vi "SUPPORTFileInitialization.vi"(11 "Camera Info":T4) -> (0 "AutonArray":dbl[][](array[numeric]), 1 "Current Auton File":string, 2 "ShooterArray":dbl[][](array[numeric]) format="%0.3f", 3 "ShooterFile":string, 4 "Number of Auton Files":i64, 5 "Auton Files":string[](array[string]))   [LabVIEW 2011]
uses:
  <vilib>/Rock Robotics/WPI/Camera/WPI_CameraImageSize.ctl
  <vilib>/Rock Robotics/WPI/Camera/WPI_CameraWhite Balance Values.ctl
  <vilib>/Rock Robotics/WPI/Camera/WPI_CameraExposure Values.ctl
  <vilib>/Utility/file.llb/Read From Spreadsheet File (DBL).vi
panel:
  out "Path and file":string
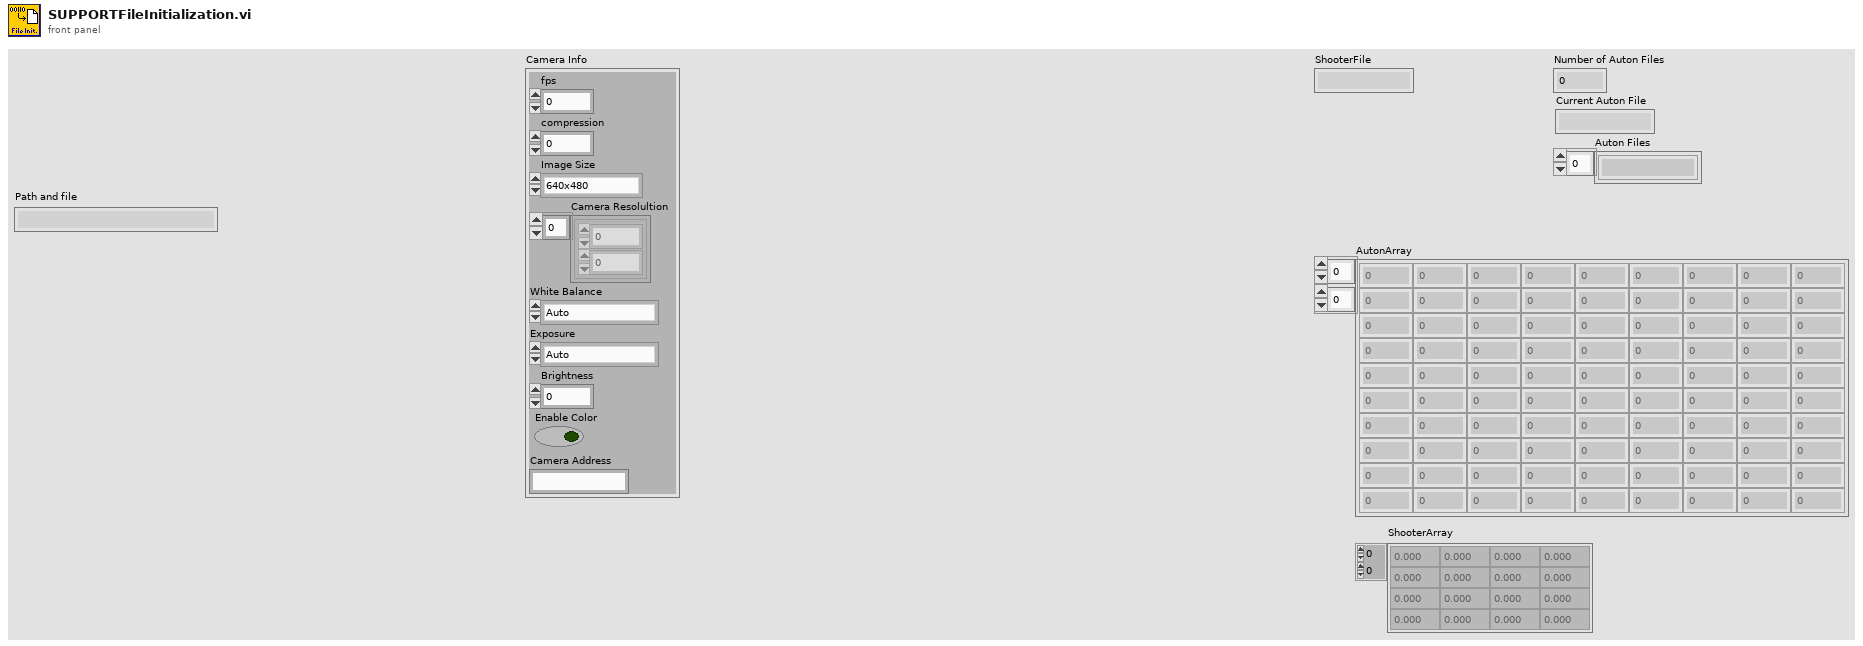
[diagram p1: front panel]
types:
  T1 = typedef "WPI_CameraImageSize.ctl" = enum16{"640x480", "320x240", "160x120"}
  T2 = typedef "WPI_CameraWhite Balance Values.ctl" = enum16{"Auto", "Fixed indoor", "Fixed outdoor 1", "Fixed outdoor 2", "Fixed fluorescent 1", "Fixed fluorescent 2", "Hold current"}
  T3 = typedef "WPI_CameraExposure Values.ctl" = enum16{"Auto", "Flicker-free 50 Hz", "Flicker-free 60 Hz", "Hold current"}
  T4 = cluster{"fps":i32, "compression":i32, "Image Size":T1, "Camera Resolultion":cluster{i32, i32}[], "White Balance":T2, "Exposure":T3, "Brightness":dbl, "Enable Color":bool, "Camera Address":string}
  T5 = typedef "WPI_CameraDevRef.ctl" = cluster{"Camera Address":string, "CameraStatus":errorcluster, "Acquire Image Notifier":refnum<notifier>}
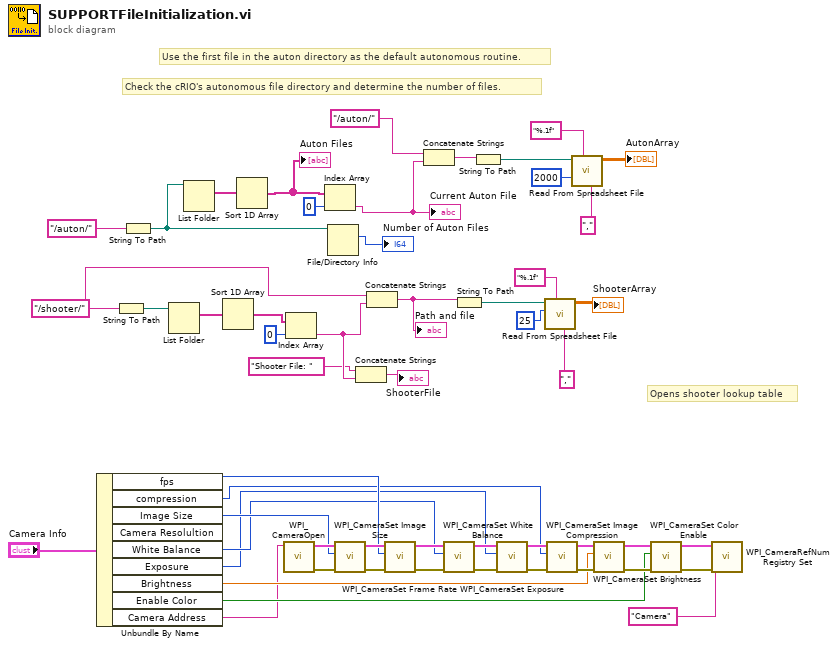
[diagram p0: block diagram]
diagram:
  w19 = "/shooter/" ("string")
  # "Check the cRIO's autonomous file directory and determine the number of files."
  # "Use the first file in the auton directory as the default autonomous routine."
  # "Opens shooter lookup table"
  n1 = Unbundle By Name("Camera Info") -> ("fps"=w37:i32, "compression"=w34:i32, "Image Size"=w38:T1, "White Balance"=w36:T2, "Exposure"=w35:T3, "Brightness"=w33:dbl, "Enable Color"=w32:bool, "Camera Address"=w31:string)  [unwired: 1 out]
  n2 = String To Path(string=w19) -> (path=w28:path)
  n3 = String To Path(string="/auton/") -> (path=w12:path)
  n4 = List Folder(path=w28) -> (filenames=w27:string[])  [unwired: 1 in, 5 out]
  n5 = List Folder(path=w12) -> (filenames=w11:string[])  [unwired: 1 in, 5 out]
  n6 = Sort 1D Array(array=w27) -> (sorted array=w26:string[])
  n7 = Sort 1D Array(array=w11) -> (sorted array=w9:string[])
  "Auton Files" <- w9
  n8 = call <vilib>:"WPI_CameraOpen.vi"("Camera Address"=w31) -> ("error out"=w45:errorcluster, "CameraDevRef"=w44:T5)  [unwired: 1 in, 8 out]
  n9 = Index Array(array=w26, index=0) -> (element=w18:string)
  n10 = Index Array(array=w9, index=0) -> (element=w1:string)
  "Current Auton File" <- w1
  n11 = File/Directory Info(path=w12) -> (size=→"Number of Auton Files":i64)  [unwired: 1 in, 6 out]
  n12 = call <vilib>:"WPI_CameraSet Image Size.vi"("error in (no error)"=w45, "Image Size"=w38, "CameraDevRef"=w44) -> ("error out"=w46:errorcluster, "CameraDevRef Out"=w43:T5)  [unwired: 7 out]
  n13 = Concatenate Strings("Shooter File: ", w18) -> (→"ShooterFile":string)
  n14 = Concatenate Strings(w19, w18) -> (w21:string)
  "Path and file" <- w21
  n15 = call <vilib>:"WPI_CameraSet Frame Rate.vi"("error in (no error)"=w46, "Frame Rate (fps)"=w37, "CameraDevRef"=w43) -> ("error out"=w47:errorcluster, "CameraDevRef Out"=w41:T5)  [unwired: 7 out]
  n16 = Concatenate Strings("/auton/" ("string"), w1) -> (w5:string)
  n17 = call <vilib>:"WPI_CameraSet White Balance.vi"("error in (no error)"=w47, "White Balance"=w36, "CameraDevRef"=w41) -> ("error out"=w48:errorcluster, "CameraDevRef Out"=w42:T5)  [unwired: 7 out]
  n18 = String To Path(string=w21) -> (path=w20:path)
  n19 = String To Path(string=w5) -> (path=w4:path)
  n20 = call <vilib>:"WPI_CameraSet Exposure.vi"("error in (no error)"=w48, "Exposure"=w35, "CameraDevRef"=w42) -> ("error out"=w49:errorcluster, "CameraDevRef Out"=w39:T5)  [unwired: 7 out]
  n21 = call-poly <vilib>:"Read From Spreadsheet File.vi"("delimiter (\\t)"="," ("delimiter (\\t)"), "format (%.3f)"="%.1f", "number of rows (all:-1)"=25, "file path (dialog if empty)"=w20) -> ("all rows"=→"ShooterArray":dbl[][])  [unwired: 1 in, 6 out]
  n22 = call <vilib>:"WPI_CameraSet Image Compression.vi"("error in (no error)"=w49, "Compression"=w34, "CameraDevRef"=w39) -> ("error out"=w50:errorcluster, "CameraDevRef Out"=w40:T5)  [unwired: 7 out]
  n23 = call-poly <vilib>:"Read From Spreadsheet File.vi"("delimiter (\\t)"="," ("delimiter (\\t)"), "format (%.3f)"="%.1f", "number of rows (all:-1)"=2000, "file path (dialog if empty)"=w4) -> ("all rows"=→"AutonArray":dbl[][])  [unwired: 1 in, 6 out]
  n24 = call <vilib>:"WPI_CameraSet Brightness.vi"("error in (no error)"=w50, "Brightness"=w33, "CameraDevRef"=w40) -> ("error out"=w52:errorcluster, "CameraDevRef Out"=w51:T5)  [unwired: 7 out]
  n25 = call <vilib>:"WPI_CameraSet Color Enable.vi"("error in (no error)"=w52, "Color Enabled"=w32, "CameraDevRef"=w51) -> ("error out"=w54:errorcluster, "CameraDevRef Out"=w53:T5)  [unwired: 7 in]
  n26 = call <vilib>:"WPI_CameraRefNum Registry Set.vi"("error in (no error)"=w54, "refnum name"="Camera", "CameraDevRef"=w53) -> ()  [unwired: 9 out]
